vi "日志、报警信息存储 (子VI).vi"   [LabVIEW 2016, in "科盛超标留样.lvlib"]
types:
  T1 = cluster{"时间标识":timestamp, "设备":string, "日志信息":string, "流程参数":string}
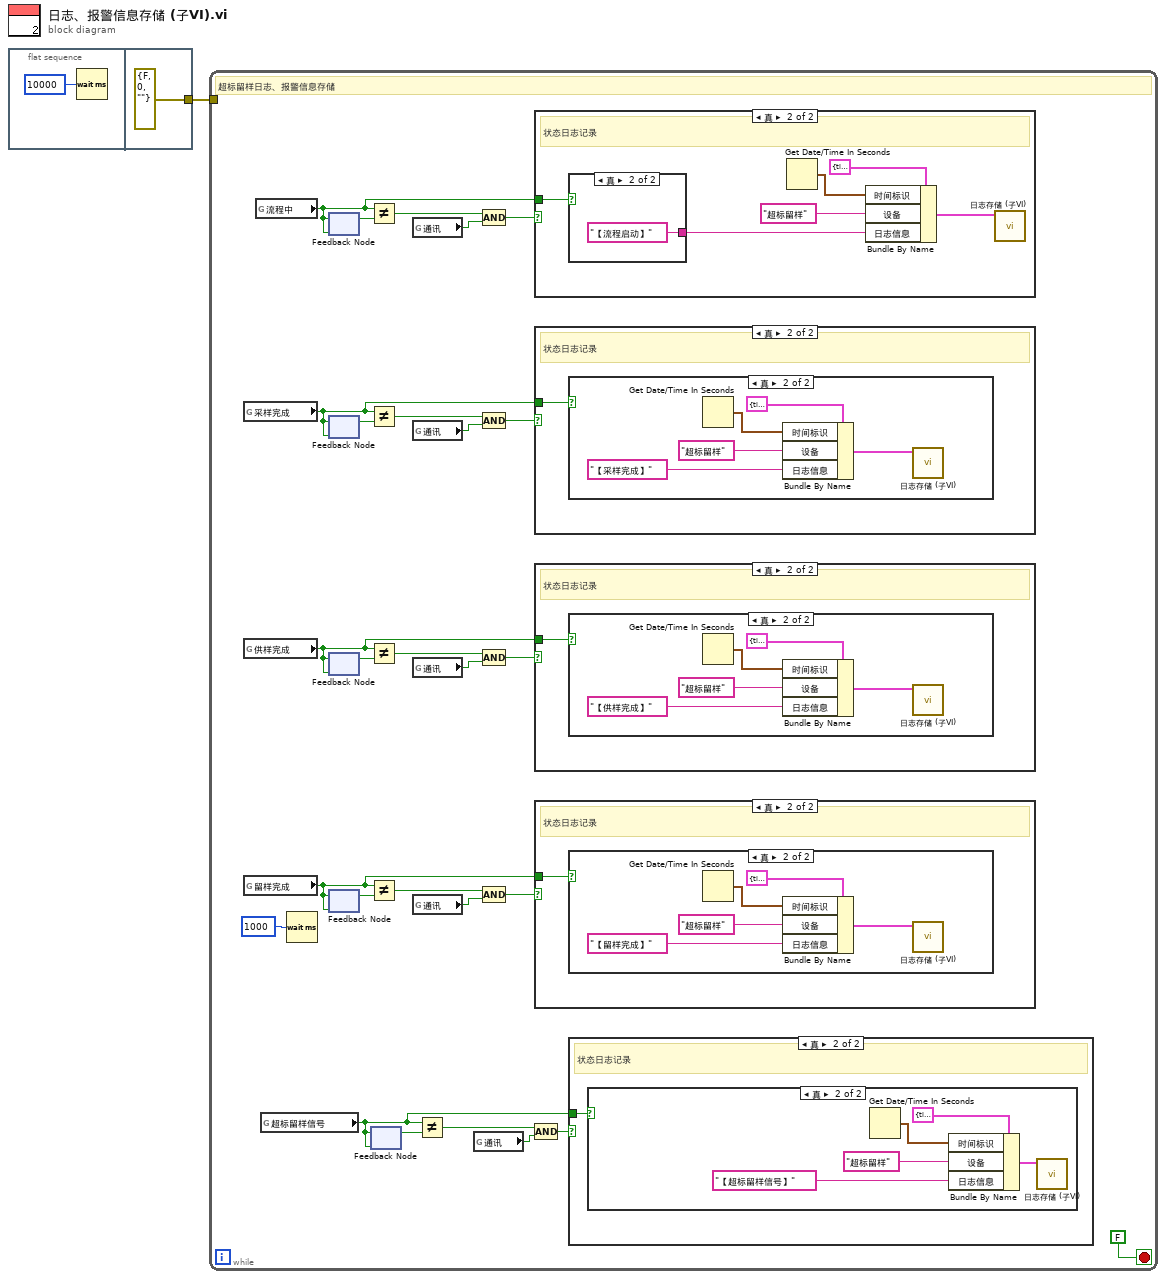
[diagram p0: block diagram]
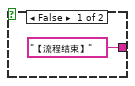
[diagram p11: hidden frame]
diagram:
  n1 = flat-sequence {
    tunnel: [errorcluster {"status"=FALSE, "code"=0, "source"=""} ("错误常量")] -> w1
    frame #0 {
      n2 = Wait (ms)(milliseconds to wait=u32 10000 ("等待时间（毫秒）")) -> ()  [unwired: 1 out]
    }
    frame #1 {
    }
  }
  n3 = while {
    tunnel: w1 -> [_]
    stop <- FALSE stop-if-true
    # "超标留样日志、报警信息存储"
    n4 = global read "超标留样全局.vi" "采样完成"() -> (w20:bool)
    n5 = global read "超标留样全局.vi" "供样完成"() -> (w19:bool)
    n6 = global read "超标留样全局.vi" "留样完成"() -> (w10:bool)
    n7 = global read "超标留样全局.vi" "流程中"() -> (w25:bool)
    n8 = global read "超标留样全局.vi" "超标留样信号"() -> (w5:bool)
    n9 = Wait (ms)(milliseconds to wait=u32 1000 ("等待时间（毫秒）")) -> ()  [unwired: 1 out]
    n10 = feedback #1(w25) -> (w29:bool)
    n11 = feedback-in #1(w25) -> ()
    n12 = feedback #2(w20) -> (w22:bool)
    n13 = feedback-in #2(w20) -> ()
    n14 = feedback #3(w19) -> (w17:bool)
    n15 = feedback-in #3(w19) -> ()
    n16 = feedback #4(w10) -> (w12:bool)
    n17 = feedback-in #4(w10) -> ()
    n18 = Not Equal?(x=w25, y=w29) -> (x != y?=w28:bool)
    n19 = Not Equal?(x=w20, y=w22) -> (x != y?=w23:bool)
    n20 = Not Equal?(x=w19, y=w17) -> (x != y?=w16:bool)
    n21 = Not Equal?(x=w10, y=w12) -> (x != y?=w13:bool)
    n22 = feedback #5(w5) -> (w8:bool)
    n23 = feedback-in #5(w5) -> ()
    n24 = global read "超标留样全局.vi" "通讯"() -> (w27:bool)
    n25 = global read "超标留样全局.vi" "通讯"() -> (w24:bool)
    n26 = global read "超标留样全局.vi" "通讯"() -> (w15:bool)
    n27 = global read "超标留样全局.vi" "通讯"() -> (w14:bool)
    n28 = Not Equal?(x=w5, y=w8) -> (x != y?=w7:bool)
    n29 = global read "超标留样全局.vi" "通讯"() -> (w6:bool)
    n30 = Compound Arithmetic op=AND ("复合运算")(w28, w27) -> (w26:bool)
    n31 = Compound Arithmetic op=AND ("复合运算")(w23, w24) -> (w21:bool)
    n32 = Compound Arithmetic op=AND ("复合运算")(w16, w15) -> (w18:bool)
    n33 = Compound Arithmetic op=AND ("复合运算")(w13, w14) -> (w11:bool)
    n34 = case shown="真" w26 {
      tunnel: w25 -> [_ w56]
      frame False {
      }
      frame True {
        # "状态日志记录"
        n35 = case shown="真" w56 {
          tunnel: ["【流程结束】" ("日志信息") "【流程启动】" ("日志信息")] -> w55
          frame False {
          }
          frame True {
          }
        }
        n36 = Get Date/Time In Seconds() -> (seconds since 1Jan1904=w59:timestamp)
        n37 = Bundle By Name(cluster=T1 {"时间标识"=timestamp(0 s since 1904-01-01), "设备"="", "日志信息"="", "流程参数"=""} ("data in"), "时间标识"=w59, "设备"="超标留样", "日志信息"=w55) -> (w58:T1)
        n38 = call "日志存储 (子VI).vi"("data in"=w58) -> ()  [unwired: 11 in]
      }
    }
    n39 = case shown="真" w21 {
      tunnel: w20 -> [_ w49]
      frame False {
      }
      frame True {
        # "状态日志记录"
        n40 = case shown="真" w49 {
          frame False {
          }
          frame True {
            n41 = Get Date/Time In Seconds() -> (seconds since 1Jan1904=w53:timestamp)
            n42 = Bundle By Name(cluster=T1 {"时间标识"=timestamp(0 s since 1904-01-01), "设备"="", "日志信息"="", "流程参数"=""} ("data in"), "时间标识"=w53, "设备"="超标留样", "日志信息"="【采样完成】") -> (w50:T1)
            n43 = call "日志存储 (子VI).vi"("data in"=w50) -> ()  [unwired: 11 in]
          }
        }
      }
    }
    n44 = case shown="真" w18 {
      tunnel: w19 -> [_ w43]
      frame False {
      }
      frame True {
        # "状态日志记录"
        n45 = case shown="真" w43 {
          frame False {
          }
          frame True {
            n46 = Get Date/Time In Seconds() -> (seconds since 1Jan1904=w47:timestamp)
            n47 = Bundle By Name(cluster=T1 {"时间标识"=timestamp(0 s since 1904-01-01), "设备"="", "日志信息"="", "流程参数"=""} ("data in"), "时间标识"=w47, "设备"="超标留样", "日志信息"="【供样完成】") -> (w44:T1)
            n48 = call "日志存储 (子VI).vi"("data in"=w44) -> ()  [unwired: 11 in]
          }
        }
      }
    }
    n49 = case shown="真" w11 {
      tunnel: w10 -> [_ w37]
      frame False {
      }
      frame True {
        # "状态日志记录"
        n50 = case shown="真" w37 {
          frame False {
          }
          frame True {
            n51 = Get Date/Time In Seconds() -> (seconds since 1Jan1904=w41:timestamp)
            n52 = Bundle By Name(cluster=T1 {"时间标识"=timestamp(0 s since 1904-01-01), "设备"="", "日志信息"="", "流程参数"=""} ("data in"), "时间标识"=w41, "设备"="超标留样", "日志信息"="【留样完成】") -> (w38:T1)
            n53 = call "日志存储 (子VI).vi"("data in"=w38) -> ()  [unwired: 11 in]
          }
        }
      }
    }
    n54 = Compound Arithmetic op=AND ("复合运算")(w7, w6) -> (w9:bool)
    n55 = case shown="真" w9 {
      tunnel: w5 -> [_ w31]
      frame False {
      }
      frame True {
        # "状态日志记录"
        n56 = case shown="真" w31 {
          frame False {
          }
          frame True {
            n57 = Get Date/Time In Seconds() -> (seconds since 1Jan1904=w35:timestamp)
            n58 = Bundle By Name(cluster=T1 {"时间标识"=timestamp(0 s since 1904-01-01), "设备"="", "日志信息"="", "流程参数"=""} ("data in"), "时间标识"=w35, "设备"="超标留样", "日志信息"="【超标留样信号】") -> (w32:T1)
            n59 = call "日志存储 (子VI).vi"("data in"=w32) -> ()  [unwired: 11 in]
          }
        }
      }
    }
  }
